vi "FPGA.vi"() -> ()   [LabVIEW 2020]
uses:
  <vilib>/rvi/Emulation/niFpgaGetClockAttributes.vi
  <vilib>/rvi/Emulation/niFpgaSctlEmulationGetInTimedLoop.vi
  <vilib>/rvi/Emulation/niFpgaEmulationReportErrorSimple.vi
  <vilib>/rvi/eio/common/nirviEmuTemplateMethod_errors.vi
  <vilib>/rvi/interface/RandomDataEmulation/niFpgaRandomDataHandleErrors.vi
  <vilib>/rvi/Emulation/niFpgaCriticalErrorInLSC.vi
  <vilib>/eio/EIONode/EIONode.xnode
  <vilib>/rvi/DataTransferAndStorage/Container/XNode/niFpgaContainer.xnode
  <vilib>/rvi/interface/RandomDataEmulation/nirviRandomDataFpgaReadWriteTemplate.vi
panel:
  out "FPGA I/O Out":refnum<k21>
  in  "Rate (uSec) 3":u32 caption="Count(uSec)"
  out "Actual loop rate 2":u32
  out "Timed Out? 3":bool
  in  "Rate (uSec) 2":u32 caption="Count(uSec)"
  out "Timed Out? 2":bool
  out "Timed Out?":bool
  out "Actual loop rate":u32
  in  "Rate (uSec)":u32 caption="Count(uSec)"
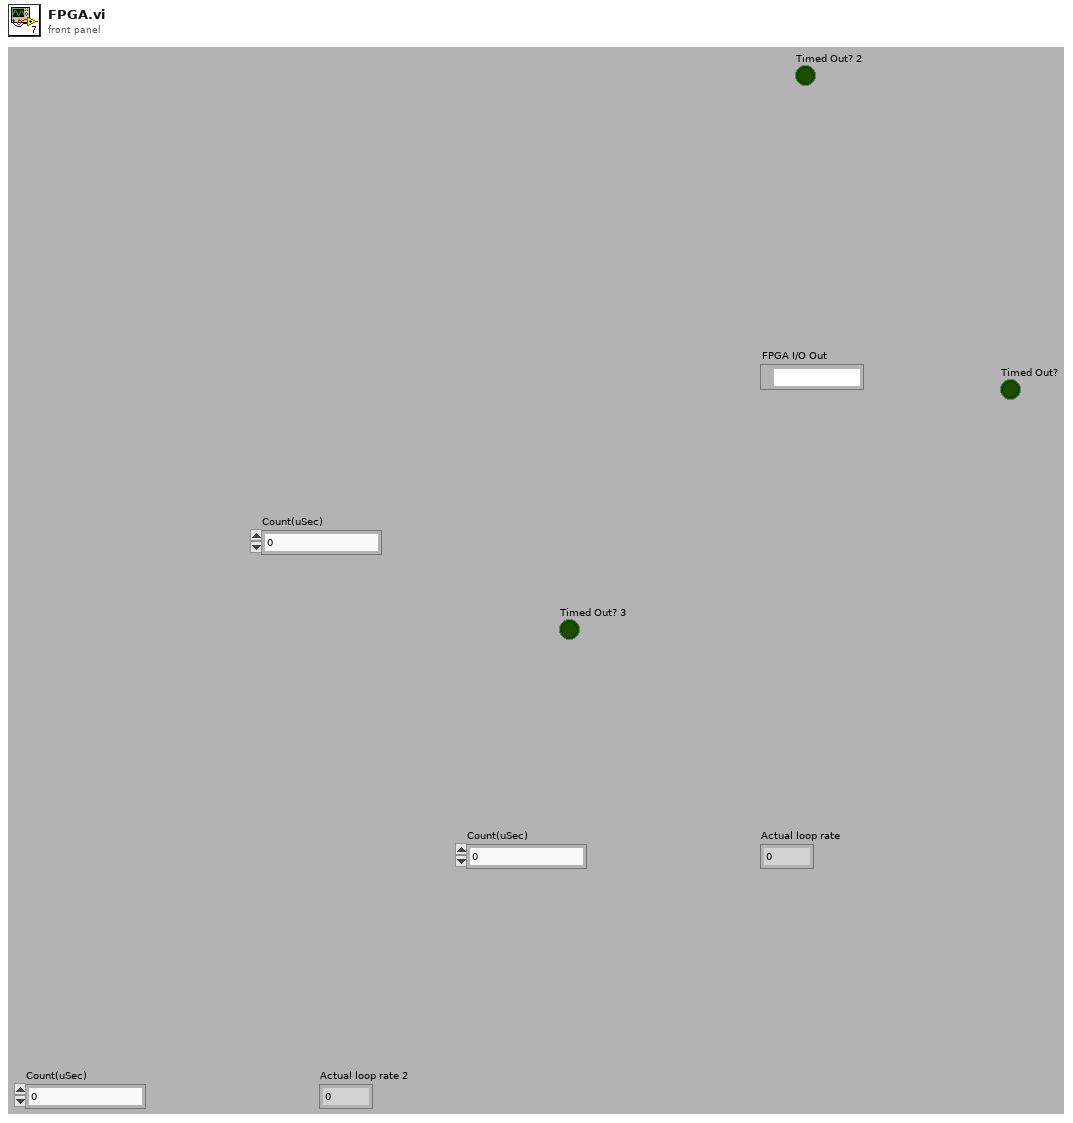
[diagram p1: front panel]
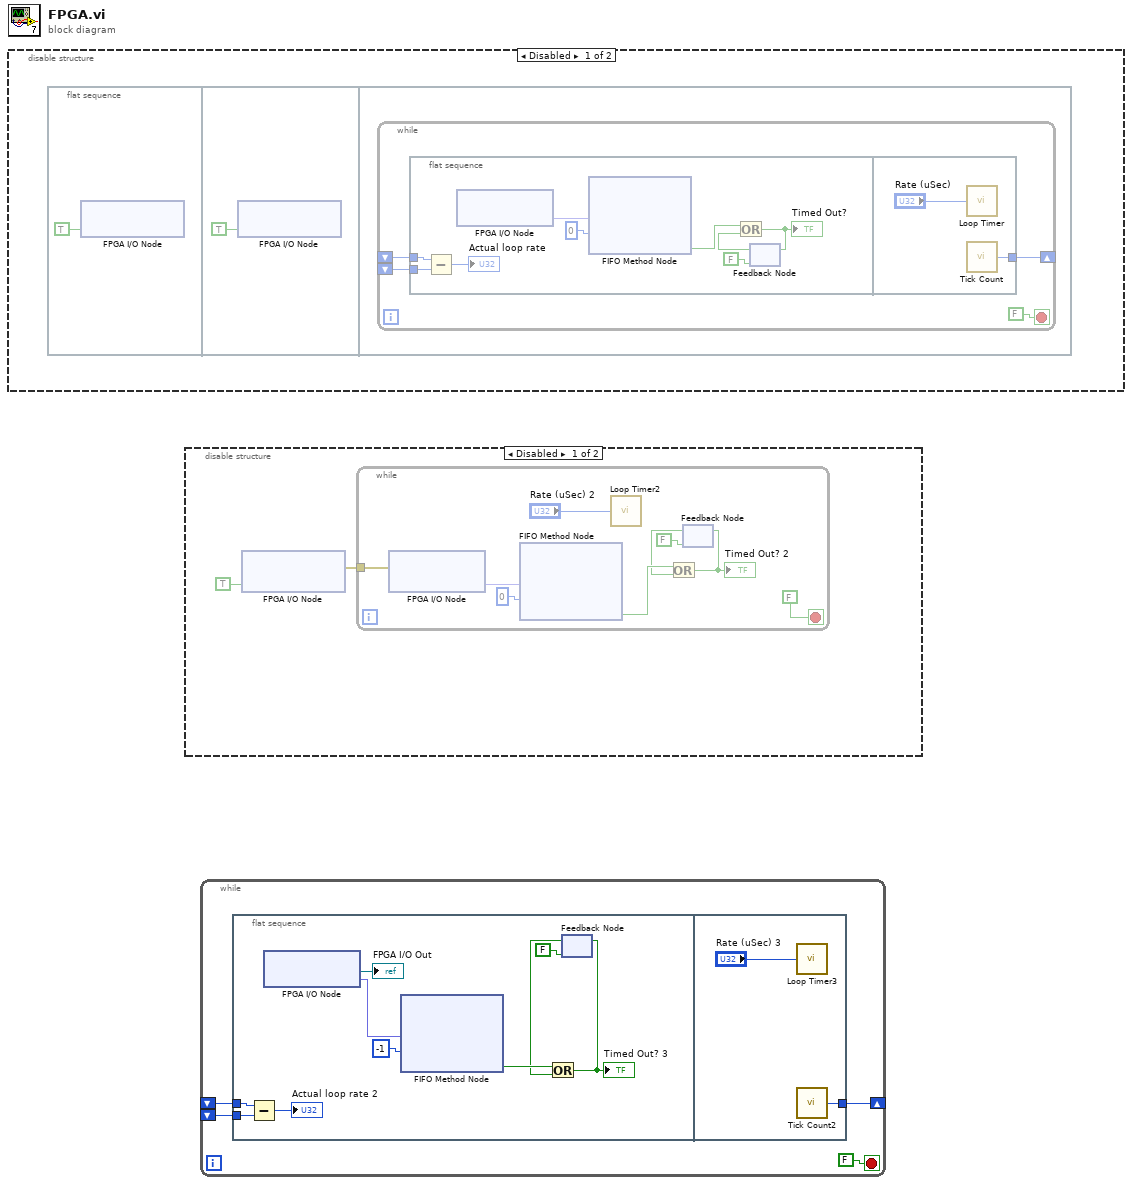
[diagram p0: block diagram]
diagram:
  n1 = disable-structure shown="Disabled" {
    frame Disabled {
      n2 = flat-sequence {
        frame #0 {
          n3 = xnode "FPGA I/O Node"("Mod1/Stop"=TRUE) -> ()  [unwired: 1 in, 1 out]
        }
        frame #1 {
          n4 = xnode "FPGA I/O Node"("Mod1/Start"=TRUE) -> ()  [unwired: 1 in, 1 out]
        }
        frame #2 {
          n5 = while {
            shift-right: [w5] -> _
            shift-left: _ -> [w4]
            shift-left: _ -> [w3]
            stop <- FALSE stop-if-true
            n6 = flat-sequence {
              tunnel: w4 -> [w15]
              tunnel: w3 -> [w14]
              tunnel: [w16] -> w5
              frame #0 {
                n7 = Subtract(x=w15, y=w14) -> (x-y=→"Actual loop rate":u32)
                n8 = xnode "FPGA I/O Node"() -> ("Mod1/AI0"=w7:fxp<+/-,24,7>)  [unwired: 1 in, 1 out]
                n9 = xnode ("FIFO Method Node")("Element"=w7, "Timeout"=0) -> ("Timed Out?"=w11:bool)  [unwired: 2 in, 2 out]
                n10 = feedback #1(FALSE) -> (w10:bool)
                n11 = Or(x=w11, y=w10) -> (x .or. y?=w9:bool)
                "Timed Out?" <- w9
                n12 = feedback-in #1(w9) -> ()
              }
              frame #1 {
                n13 = call "Loop Timer"("Count(uSec)"="Rate (uSec)") -> ()  [unwired: 1 out]
                n14 = call "Tick Count"() -> ("Tick Count(uSec)"=w16:u32)
              }
            }
          }
        }
      }
    }
    frame Enabled {
    }
  }
  n15 = disable-structure shown="Disabled" {
    frame Disabled {
      n16 = xnode "FPGA I/O Node"("Mod1/Start"=TRUE) -> ("error out"=w19:errorcluster)  [unwired: 2 in, 1 out]
      n17 = while {
        tunnel: w19 -> [w27]
        stop <- FALSE stop-if-true
        n18 = xnode "FPGA I/O Node"("error in"=w27) -> ("Mod1/AI0"=w21:fxp<+/-,24,7>)  [unwired: 1 in, 2 out]
        n19 = xnode ("FIFO Method Node")("Element"=w21, "Timeout"=0) -> ("Timed Out?"=w25:bool)  [unwired: 2 in, 2 out]
        n20 = call "Loop Timer2"("Count(uSec)"="Rate (uSec) 2") -> ()  [unwired: 1 out]
        n21 = feedback #2(FALSE) -> (w24:bool)
        n22 = Or(x=w25, y=w24) -> (x .or. y?=w23:bool)
        "Timed Out? 2" <- w23
        n23 = feedback-in #2(w23) -> ()
      }
    }
    frame Enabled {
    }
  }
  n24 = while {
    shift-right: [w31] -> _
    shift-left: _ -> [w30]
    shift-left: _ -> [w29]
    stop <- FALSE stop-if-true
    n25 = flat-sequence {
      tunnel: w30 -> [w42]
      tunnel: w29 -> [w41]
      tunnel: [w43] -> w31
      frame #0 {
        n26 = Subtract(x=w42, y=w41) -> (x-y=→"Actual loop rate 2":u32)
        n27 = xnode "FPGA I/O Node"() -> ("Mod1/AI0"=w34:fxp<+/-,24,7>, "FPGA I/O Out"=→"FPGA I/O Out":refnum<k21>)  [unwired: 1 in]
        n28 = xnode ("FIFO Method Node")("Element"=w34, "Timeout"=-1) -> ("Timed Out?"=w38:bool)  [unwired: 2 in, 2 out]
        n29 = feedback #3(FALSE) -> (w37:bool)
        n30 = Or(x=w38, y=w37) -> (x .or. y?=w36:bool)
        "Timed Out? 3" <- w36
        n31 = feedback-in #3(w36) -> ()
      }
      frame #1 {
        n32 = call "Loop Timer3"("Count(uSec)"="Rate (uSec) 3") -> ()  [unwired: 1 out]
        n33 = call "Tick Count2"() -> ("Tick Count(uSec)"=w43:u32)
      }
    }
  }
